vi "Biax24X setup (16chan).vi"() -> (0 "buffer size":i32=500000, 1 "Footer String":string, 2 "Channels (1-8), Hor load, Hor Disp, Vert Load, Vert Disp, Pc Disp, Pc load, Ppa Disp, Ppa load":string[](array[string])=["0:3", "0:3", "0:3", "0:3"], 3 "Number of Channels":i32, 4 "ASCII footer 2":bool, 5 "Device":i32=2, 6 "Channel Names":string[](array[string]), 8 "Header and Const.; Del, SR, #Scans, Write int":T1={"Delay"=-1.0, "Scan_Rate"=10000, "Number of scans"=10000, "Write time int (s)"=30} {"Delay" format="%.2f"})   [LabVIEW 2013]
doc: "This vi takes input from the operator: sets the scan rate, collects the length in inches, the sample diameter in inches, and the interchannel delay rate (default is -1.0) The vi puts out those constants along with the voltage limits for each of the data acquisition channels. The default settings are channel 0, 1 = confining and pore pressure transducer amplifiers, respectively, 0-5 volts; temperature transducer amplifier, 0-5 volts; dcdt +-3 volts (12.6 v/in); load cell after amplification: 12600 pounds force per volt."
uses:
  BiaxGlobals (16chan).vi
panel:
  out "Device 2":i32=1
  in  "String 31":string="AUX 1"
  in  "String 30":string="AUX 2"
  in  "String 29":string="AUX 6"
  in  "String 28":string="AUX 5"
  in  "String 27":string="AUX 4"
  in  "String 26":string="AUX 3"
  in  "String 25":string="Ppb LOAD"
  in  "String 24":string="Ppb Disp"
  in  "ASCII footer":bool=TRUE
  in  "String 23":string="Vert DCDT"
  in  "String 22":string="Vert LOAD"
  in  "String 21":string="Hor DCDT"
  in  "String 20":string="Hor LOAD"
  in  "String 19":string="Pc Disp"
  in  "String 18":string="Pc LOAD"
  in  "String 17":string="Ppa Disp"
  in  "String 16":string="Ppa LOAD"
  in  "Number of Channels":i32=10 min=9 max=16 step=1
  in  "Go on":bool
  in  "Delay":sgl=-1.0 format="%^.2e"
  out "Acquisition Rate \n(fixed at 10000 \nsamples/sec)":i32=10000
  out "Number of scans averaged for a single record output\n(while running Labview you can switch between 1, 10, 100, 1k, 10k samples/sec)":i32=10000
  in  "buffer size (500000 scans)":i32=500000
  out "write int":i32=30
  in  "Time interval to write to disk (seconds)\nNOTE: 30sec is optimal for 10 kHz sample rate":i32=30
  # "Press \"Go On\" when\nConstants are Entered\n\nDefault Delay setting \nis -1.0"
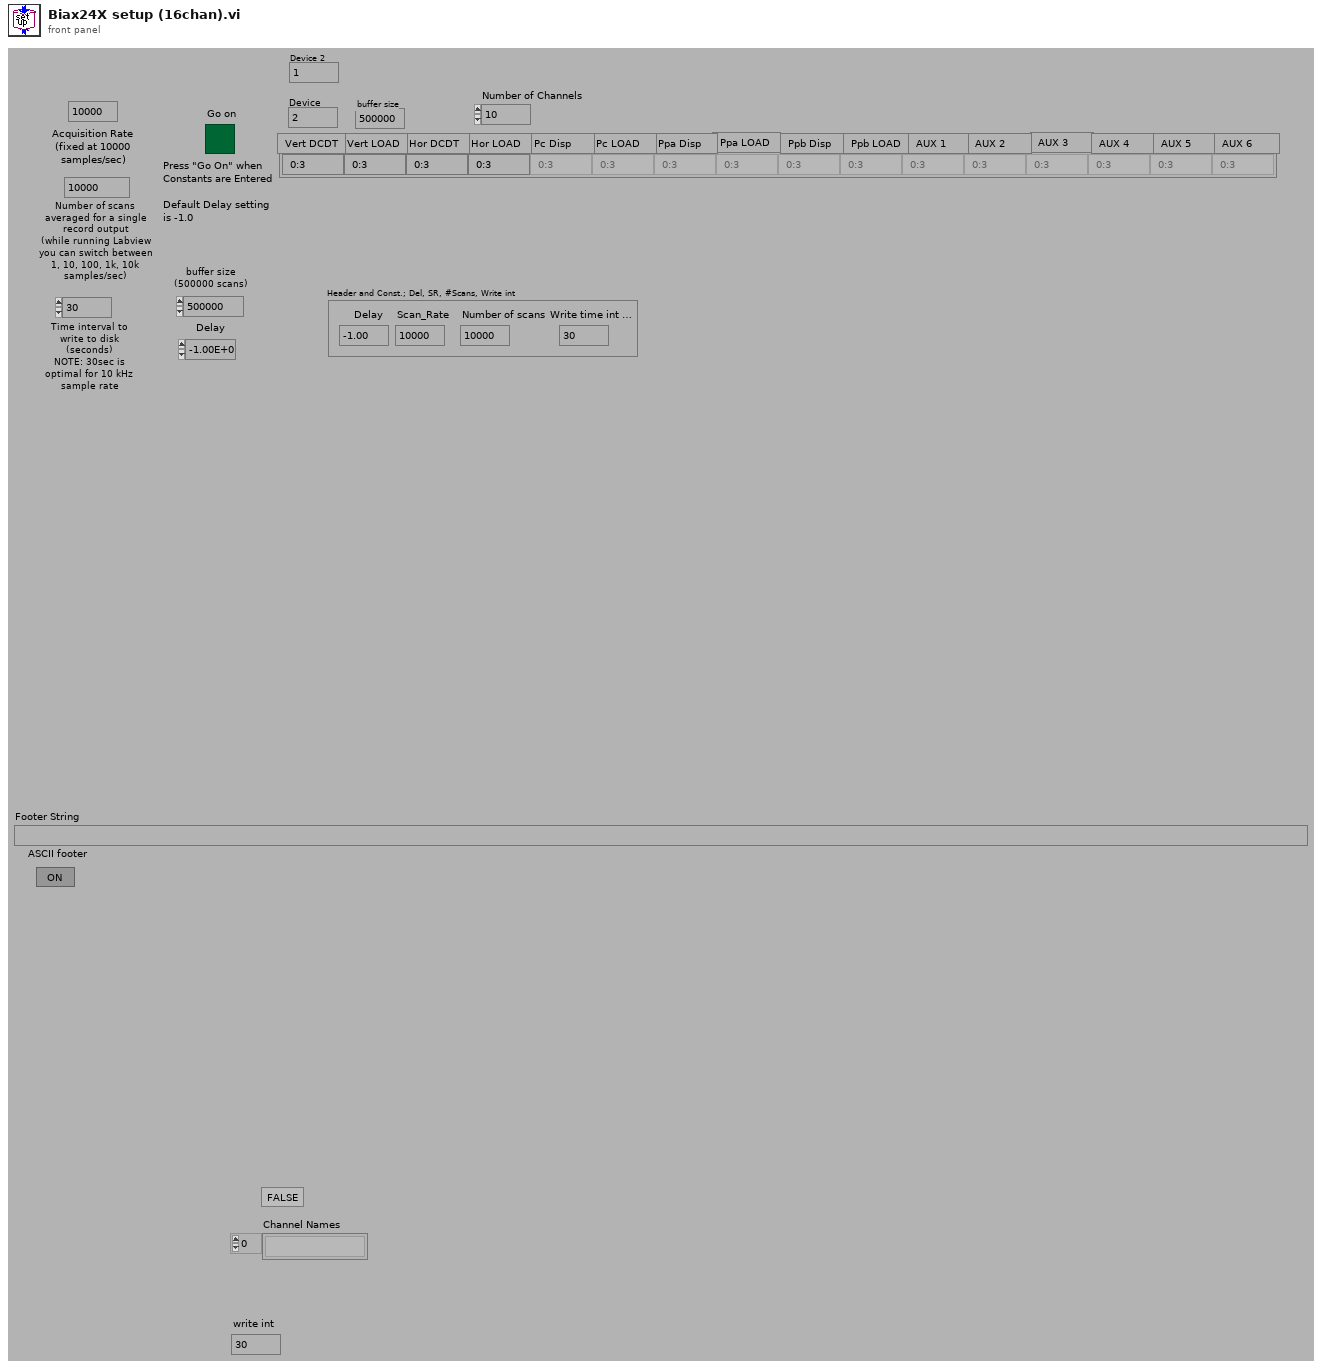
[diagram p1: front panel]
types:
  T1 = cluster{"Delay":dbl, "Scan_Rate":i32, "Number of scans":i32, "Write time int (s)":i32}
  T2 = cluster{"Delay":sgl, i32, i32, "Time interval to write to disk (seconds)\nNOTE: 30sec is optimal for 10 kHz sample rate":i32}
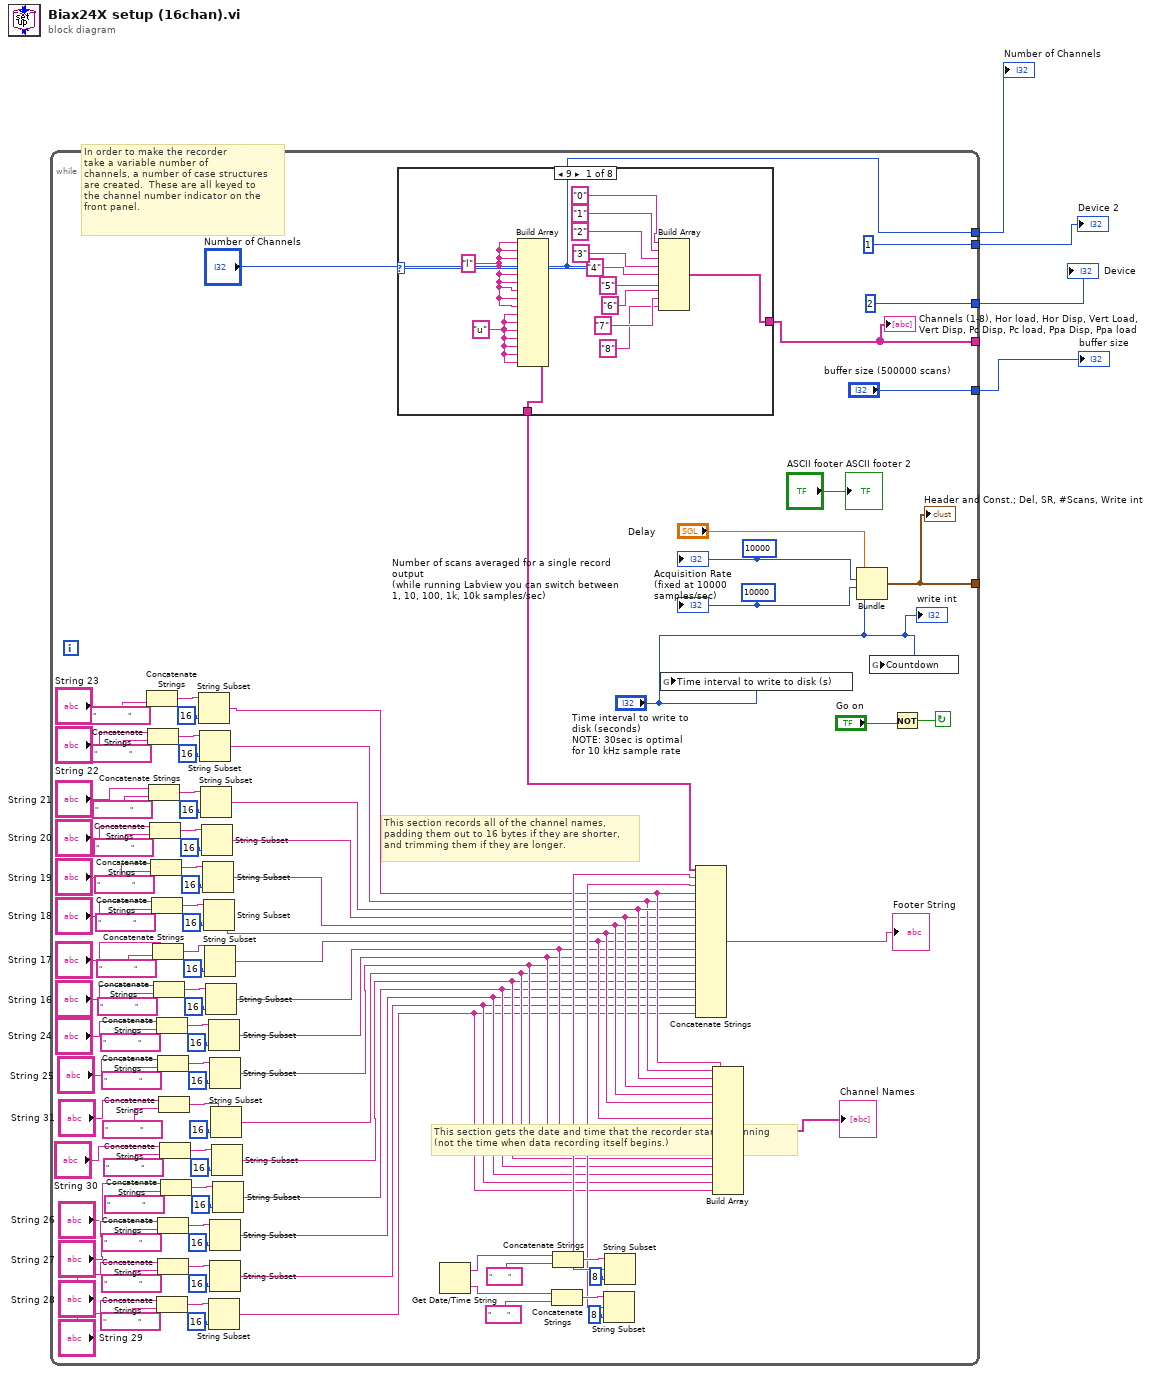
[diagram p0: block diagram]
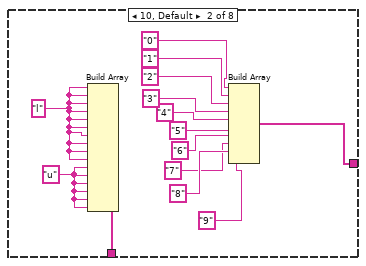
[diagram p2: hidden frame]
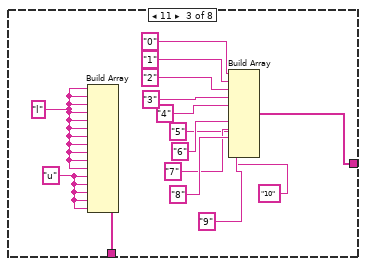
[diagram p3: hidden frame]
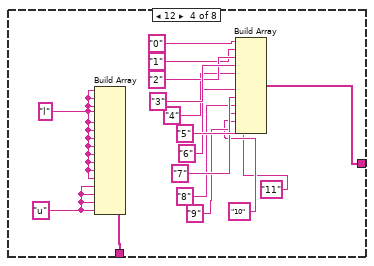
[diagram p4: hidden frame]
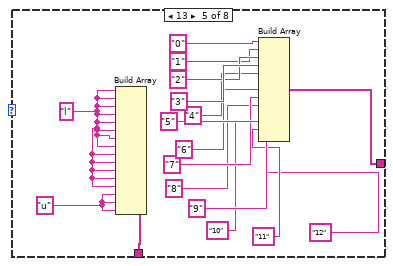
[diagram p5: hidden frame]
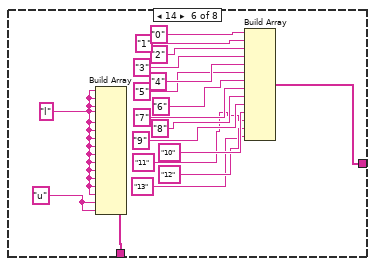
[diagram p6: hidden frame]
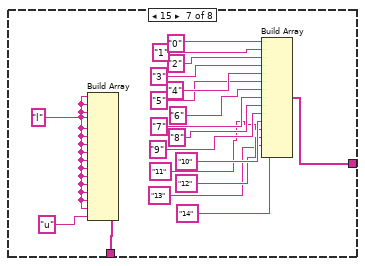
[diagram p7: hidden frame]
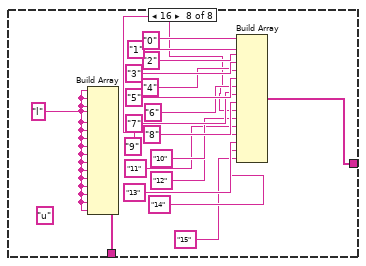
[diagram p8: hidden frame]
diagram:
  n1 = while {
    tunnel: ["buffer size (500000 scans)"] -> w4
    tunnel: [w101] -> _
    tunnel: [2] -> w3
    tunnel: [w6] -> _
    tunnel: ["Number of Channels"] -> w2
    tunnel: [1] -> w1
    stop <- w109 continue-if-true
    w103 = 10000
    w104 = 10000
    # "In order to make the recorder\ntake a variable number of\nchannels, a number of case structures\nare created.  These are all keyed to\nthe channel number indicator on the\nfront panel."
    # "This section gets the date and time that the recorder started running \n(not the time when data recording itself begins.)"
    # "This section records all of the channel names,\npadding them out to 16 bytes if they are shorter,\nand trimming them if they are longer."
    n2 = Concatenate Strings("String 23", "                ") -> (w98:string)
    n3 = Concatenate Strings("String 22", "                ") -> (w95:string)
    n4 = Concatenate Strings("String 21", "                ") -> (w92:string)
    n5 = Concatenate Strings("String 20", "                ") -> (w89:string)
    n6 = Concatenate Strings("String 19", "                ") -> (w86:string)
    n7 = Concatenate Strings("String 18", "                ") -> (w83:string)
    n8 = Concatenate Strings("String 17", "                ") -> (w80:string)
    n9 = Concatenate Strings("String 16", "                ") -> (w77:string)
    n10 = Concatenate Strings("String 24", "                ") -> (w74:string)
    n11 = Concatenate Strings("String 29", "                ") -> (w53:string)
    n12 = Concatenate Strings("String 25", "                ") -> (w71:string)
    n13 = Concatenate Strings("String 27", "                ") -> (w59:string)
    n14 = Concatenate Strings("String 28", "                ") -> (w56:string)
    n15 = Concatenate Strings("String 31", "                ") -> (w68:string)
    n16 = Concatenate Strings("String 30", "                ") -> (w65:string)
    n17 = Concatenate Strings("String 26", "                ") -> (w62:string)
    n18 = String Subset(string=w98, length (rest)=16 ("length (rest)")) -> (substring=w34:string)  [unwired: 1 in]
    n19 = String Subset(string=w95, length (rest)=16 ("length (rest)")) -> (substring=w32:string)  [unwired: 1 in]
    n20 = String Subset(string=w92, length (rest)=16 ("length (rest)")) -> (substring=w33:string)  [unwired: 1 in]
    n21 = String Subset(string=w89, length (rest)=16 ("length (rest)")) -> (substring=w31:string)  [unwired: 1 in]
    n22 = String Subset(string=w86, length (rest)=16 ("length (rest)")) -> (substring=w30:string)  [unwired: 1 in]
    n23 = String Subset(string=w83, length (rest)=16 ("length (rest)")) -> (substring=w29:string)  [unwired: 1 in]
    n24 = String Subset(string=w80, length (rest)=16 ("length (rest)")) -> (substring=w28:string)  [unwired: 1 in]
    n25 = String Subset(string=w77, length (rest)=16 ("length (rest)")) -> (substring=w27:string)  [unwired: 1 in]
    n26 = String Subset(string=w74, length (rest)=16 ("length (rest)")) -> (substring=w26:string)  [unwired: 1 in]
    n27 = String Subset(string=w53, length (rest)=16 ("length (rest)")) -> (substring=w19:string)  [unwired: 1 in]
    n28 = String Subset(string=w71, length (rest)=16 ("length (rest)")) -> (substring=w25:string)  [unwired: 1 in]
    n29 = String Subset(string=w59, length (rest)=16 ("length (rest)")) -> (substring=w21:string)  [unwired: 1 in]
    n30 = String Subset(string=w56, length (rest)=16 ("length (rest)")) -> (substring=w20:string)  [unwired: 1 in]
    n31 = String Subset(string=w68, length (rest)=16 ("length (rest)")) -> (substring=w24:string)  [unwired: 1 in]
    n32 = String Subset(string=w65, length (rest)=16 ("length (rest)")) -> (substring=w23:string)  [unwired: 1 in]
    n33 = String Subset(string=w62, length (rest)=16 ("length (rest)")) -> (substring=w22:string)  [unwired: 1 in]
    n34 = case shown="9" "Number of Channels" {
      tunnel: [w116 w127 w141 w157 w174 w193 w207 w241] -> w6
      tunnel: [w117 w126 w140 w156 w173 w192 w221 w239] -> w15
      frame 9 {
        w111 = "u" ("element")
        w112 = "l"
        n35 = Build Array(w112, w112, w112, w112, w112, w112, w112, w112, w112, w111, w111, w111, w111, w111, w111, w111) -> (w117:string[])
        n36 = Build Array("0", "1", "2", "3", "4", "5", "6", "7", "8") -> (w116:string[])
      }
      frame 10, Default {
        w124 = "u" ("element")
        w125 = "l"
        n37 = Build Array(w125, w125, w125, w125, w125, w125, w125, w125, w125, w125, w124, w124, w124, w124, w124, w124) -> (w126:string[])
        n38 = Build Array("0", "1", "2", "3", "4", "5", "6", "7", "8", "9") -> (w127:string[])
      }
      frame 11 {
        w142 = "u" ("element")
        w138 = "l"
        n39 = Build Array(w138, w138, w138, w138, w138, w138, w138, w138, w138, w138, w138, w142, w142, w142, w142, w142) -> (w140:string[])
        n40 = Build Array("0", "1", "2", "3", "4", "5", "6", "7", "8", "9", "10") -> (w141:string[])
      }
      frame 12 {
        w168 = "u" ("element")
        w153 = "l"
        n41 = Build Array(w153, w153, w153, w153, w153, w153, w153, w153, w153, w153, w153, w153, w168, w168, w168, w168) -> (w156:string[])
        n42 = Build Array("0", "1", "2", "3", "4", "5", "6", "7", "8", "9", "10", "11") -> (w157:string[])
      }
      frame 13 {
        w185 = "u" ("element")
        w169 = "l"
        n43 = Build Array(w169, w169, w169, w169, w169, w169, w169, w169, w169, w169, w169, w169, w169, w185, w185, w185) -> (w173:string[])
        n44 = Build Array("0", "1", "2", "3", "4", "5", "6", "7", "8", "9", "10", "11", "12") -> (w174:string[])
      }
      frame 14 {
        w194 = "u" ("element")
        w186 = "l"
        n45 = Build Array(w186, w186, w186, w186, w186, w186, w186, w186, w186, w186, w186, w186, w186, w186, w194, w194) -> (w192:string[])
        n46 = Build Array("0", "1", "2", "3", "4", "5", "6", "7", "8", "9", "10", "11", "12", "13") -> (w193:string[])
      }
      frame 15 {
        w204 = "l"
        n47 = Build Array(w204, w204, w204, w204, w204, w204, w204, w204, w204, w204, w204, w204, w204, w204, w204, "u" ("element")) -> (w221:string[])
        n48 = Build Array("0", "1", "2", "3", "4", "5", "6", "7", "8", "9", "10", "11", "12", "13", "14") -> (w207:string[])
      }
      frame 16 {
        (unwired) "u" ("element")
        w223 = "l"
        n49 = Build Array(w223, w223, w223, w223, w223, w223, w223, w223, w223, w223, w223, w223, w223, w223, w223, w223) -> (w239:string[])
        n50 = Build Array("0", "1", "2", "3", "4", "5", "6", "7", "8", "9", "10", "11", "12", "13", "14", "15") -> (w241:string[])
      }
    }
    "Channels (1-8), Hor load, Hor Disp, Vert Load, Vert Disp, Pc Disp, Pc load, Ppa Disp, Ppa load" <- w6
    n51 = Get Date/Time String() -> (date string=w38:string, time string=w37:string)  [unwired: 3 in]
    n52 = Concatenate Strings(w37, "        ") -> (w40:string)
    n53 = Concatenate Strings(w38, "        ") -> (w43:string)
    n54 = String Subset(string=w40, length (rest)=8 ("length (rest)")) -> (substring=w35:string)  [unwired: 1 in]
    n55 = String Subset(string=w43, length (rest)=8 ("length (rest)")) -> (substring=w36:string)  [unwired: 1 in]
    n56 = global write "BiaxGlobals (16chan).vi" "Time interval to write to disk (s)"("Time interval to write to disk (seconds)\nNOTE: 30sec is optimal for 10 kHz sample rate") -> ()
    n57 = Concatenate Strings(w15, w36, w35, w34, w32, w33, w31, w30, w29, w28, w27, w26, w25, w24, w23, w22, w21, w20, w19) -> (→"Footer String":string)
    n58 = Build Array(w34, w32, w33, w31, w30, w29, w28, w27, w26, w25, w24, w23, w22, w21, w20, w19) -> (→"Channel Names":string[])
    n59 = Bundle("Delay"="Delay", w104, w103, "Time interval to write to disk (seconds)\nNOTE: 30sec is optimal for 10 kHz sample rate"="Time interval to write to disk (seconds)\nNOTE: 30sec is optimal for 10 kHz sample rate") -> (w101:T2)  [unwired: 1 in]
    "Header and Const.; Del, SR, #Scans, Write int" <- w101
    n60 = global write "BiaxGlobals (16chan).vi" "Countdown"("Time interval to write to disk (seconds)\nNOTE: 30sec is optimal for 10 kHz sample rate") -> ()
    n61 = Not(x="Go on") -> (.not. x?=w109:bool)
    "Acquisition Rate \n(fixed at 10000 \nsamples/sec)" <- w104
    "Number of scans averaged for a single record output\n(while running Labview you can switch between 1, 10, 100, 1k, 10k samples/sec)" <- w103
    "write int" <- "Time interval to write to disk (seconds)\nNOTE: 30sec is optimal for 10 kHz sample rate"
    "ASCII footer 2" <- "ASCII footer"
  }
  "Device" <- w3
  "buffer size" <- w4
  "Number of Channels" <- w2
  "Device 2" <- w1
